vi "Main.vi"(11 "Script in":refnum<class "_Rename.lvclass">) -> ()   [LabVIEW 2021, in "_Rename.lvlib" / "_Rename.lvclass"]
uses:
  _Rename.lvclass
  _Rename.lvclass/_Rename.ctl
  <vilib>/Utility/EditLVLibs/Edit LVLibs.lvlib
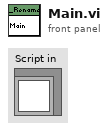
[diagram p1: front panel]
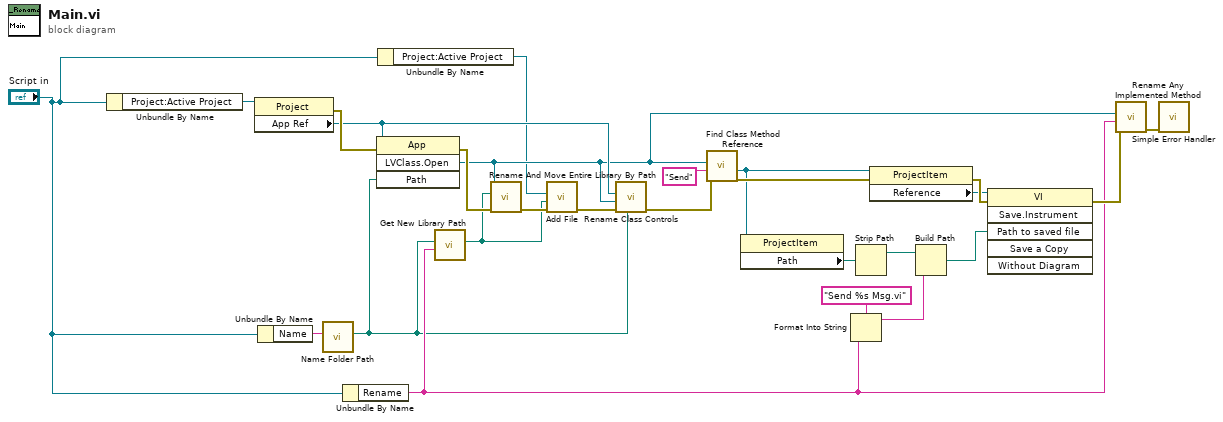
[diagram p0: block diagram]
diagram:
  n1 = Unbundle By Name("Script in") -> ("Project:Active Project"=w6:refnum<vi>)
  n2 = property class="Project"(reference=w6) -> (error out=w24:errorcluster, "App Ref"=w10:refnum<vi>)  [unwired: 1 in, 1 out]
  n3 = Unbundle By Name("Script in") -> ("Name"=w2:string)
  n4 = call "Name Folder Path.vi"("Name"=w2) -> ("Name Folder Path"=w1:path)  [unwired: 10 in]
  n5 = Unbundle By Name("Script in") -> ("Rename"=w3:string)
  n6 = invoke class="App" method="LVClass.Open"(reference=w10, error in=w24, "Path"=w1) -> (error out=w25:errorcluster, "LVClass.Open"=w8:refnum<vi>)  [unwired: 1 in, 2 out]
  n7 = Unbundle By Name("Script in") -> ("Project:Active Project"=w5:refnum<vi>)
  n8 = call "Get New Library Path.vi"("Rename"=w3, "Name Folder Path"=w1) -> ("New Library Path"=w9:path)  [unwired: 9 in]
  n9 = call <vilib>:"Rename And Move Entire Library By Path.vi"("error in (no error)"=w25, "New library path"=w9, "Library ref in"=w8) -> ("error out"=w11:errorcluster)  [unwired: 7 in, 1 out]
  n10 = call "Add File.vi"("error in"=w11, "Path"=w9, "Project:Active Project"=w5) -> ("error out"=w7:errorcluster)  [unwired: 8 in]
  n11 = call "Rename Class Controls.vi"("Old Class"=w1, "error in"=w7, "Class To Rename"=w8, "Application Instance"=w10) -> ("error out"=w16:errorcluster)  [unwired: 7 in]
  n12 = call "Find Class Method Reference.vi"("error in"=w16, "Method Name"="Send" ("regular expression"), "Class To Rename"=w8) -> ("error out"=w15:errorcluster, "Method Reference"=w12:refnum<vi>)  [unwired: 7 in]
  n13 = property class="ProjectItem"(reference=w12) -> ("Path"=w18:path)  [unwired: 1 in, 2 out]
  n14 = Format Into String(format string="Send %s Msg.vi", w3) -> (resulting string=w13:string)  [unwired: 2 in, 1 out]
  n15 = Strip Path(path=w18) -> (stripped path=w23:path)  [unwired: 1 out]
  n16 = property class="ProjectItem"(reference=w12, error in=w15) -> (error out=w26:errorcluster, "Reference"=w22:refnum<vi>)  [unwired: 1 out]
  n17 = Build Path(base path=w23, name or relative path=w13) -> (appended path=w21:path)
  n18 = invoke class="VI" method="Save.Instrument"(reference=w22, error in=w26, "Path to saved file"=w21) -> (error out=w19:errorcluster)  [unwired: 3 in, 5 out]
  n19 = call "Rename Any Implemented Method.vi"("error in"=w19, "Name"=w3, "Class To Rename"=w8) -> ("error out"=w20:errorcluster)  [unwired: 8 in]
  n20 = call <vilib>:"Simple Error Handler.vi"("error in (no error)"=w20) -> ()  [unwired: 4 in, 5 out]
